vi "Calc Stat.vi"(9 "Query Parameters":T1, 11 "Channel Data":dbl[](array[numeric])) -> (0 "Maximum":dbl, 1 "Variance":dbl, 2 "Standard Deviation":dbl, 3 "Mean":dbl, 4 "Minimum":dbl, 5 "Median":dbl, 6 "N":dbl)   [LabVIEW 2011]
uses:
  Datasheet Analysis Parameters.ctl
  <vilib>/Analysis/NI_AALBase.lvlib
panel:
  # "DELAY format data must be calculated prior to passing to this VI"
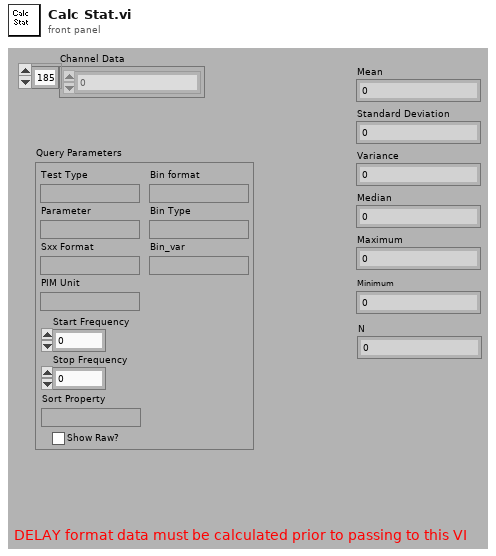
[diagram p1: front panel]
types:
  T1 = typedef "Datasheet Analysis Parameters.ctl" = cluster{"Test Type":string, "Parameter":string, "Sxx Format":string, "PIM Unit":string, "Start Frequency":dbl, "Stop Frequency":dbl, "Sort Property":string, "Show Raw?":bool, "Bin format":string, "Bin Type":string, "Bin_var":string}
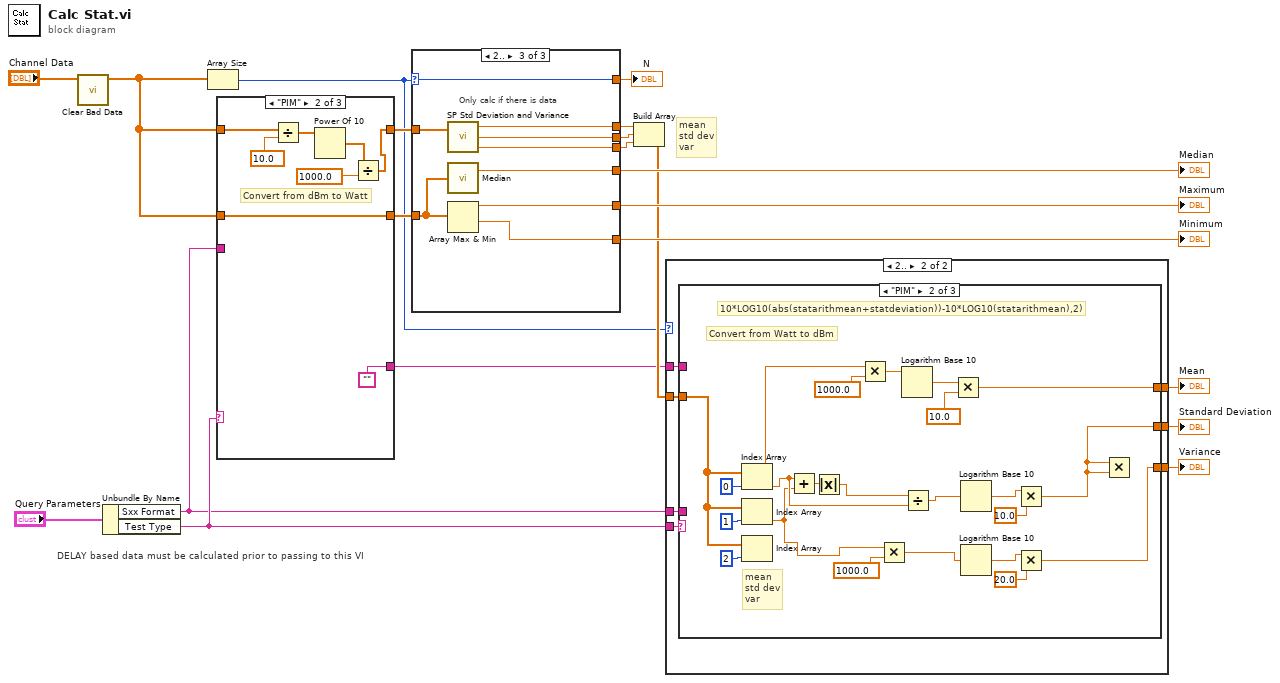
[diagram p0: block diagram]
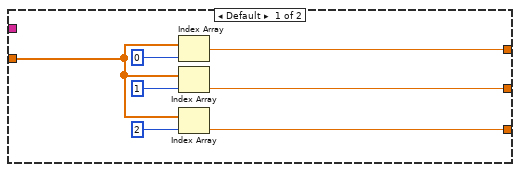
[diagram p2: hidden frame]
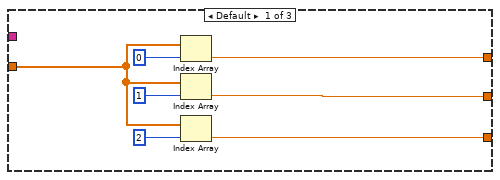
[diagram p3: hidden frame]
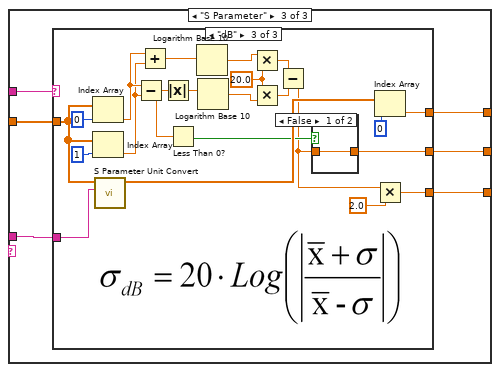
[diagram p4: hidden frame]
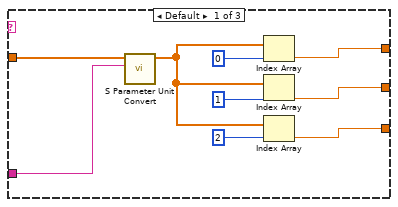
[diagram p5: hidden frame]
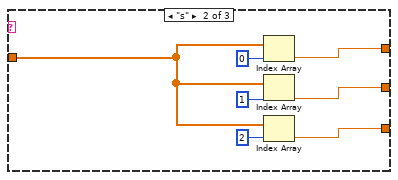
[diagram p6: hidden frame]
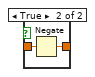
[diagram p7: hidden frame]
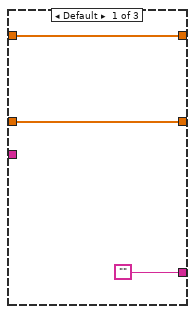
[diagram p8: hidden frame]
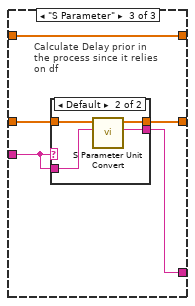
[diagram p9: hidden frame]
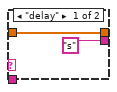
[diagram p10: hidden frame]
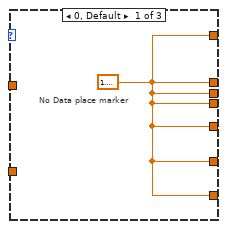
[diagram p11: hidden frame]
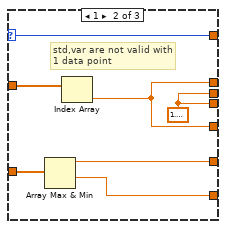
[diagram p12: hidden frame]
diagram:
  # "mean\nstd dev\nvar"
  # "DELAY based data must be calculated prior to passing to this VI"
  n1 = call "Clear Bad Data.vi"("Waveform IN"="Channel Data") -> ("Waveform out"=w3:dbl[])  [unwired: 10 out]
  n2 = Unbundle By Name("Query Parameters") -> ("Sxx Format"=w15:string, "Test Type"=w16:string)
  n3 = Array Size(array=w3) -> (size(s)=w2:i32)
  n4 = case shown="\"PIM\"" w16 {
    tunnel: w3 -> [w23 w26 w36]
    tunnel: [w23 w26 w35] -> w14
    tunnel: w15 -> [_ _ w33]
    tunnel: ["" "" w34] -> w6
    tunnel: [w21 w24 w32] -> w4
    tunnel: w3 -> [w21 w27 w32]
    frame Default {
    }
    frame "PIM" {
      # "Convert from dBm to Watt"
      n5 = Divide(x=w27, y=10.0) -> (x/y=w28:dbl[])
      n6 = Power Of 10(x=w28) -> (10^x=w29:dbl[])
      n7 = Divide(x=w29, y=1000.0) -> (x/y=w24:dbl[])
    }
    frame "S Parameter" {
      # "Calculate Delay prior in the process since it relies on df"
      n8 = case shown="Default" w33 {
        tunnel: w36 -> [w38 w42]
        tunnel: [w38 w41] -> w35
        tunnel: w33 -> [_ w40]
        tunnel: ["s" w39] -> w34
        frame "delay" {
        }
        frame Default {
          n9 = call "S Parameter Unit Convert.vi"("Format"=w40, "Waveform IN"=w42) -> ("Units"=w39:string, "Waveform out"=w41:dbl[])  [unwired: 1 in, 7 out]
        }
      }
    }
  }
  n10 = case shown="2.." w2 {
    selector: w2 -> [_ w44 w53]
    tunnel: [w43 w45 w59] -> w19
    tunnel: [w43 w47 w58] -> w18
    tunnel: [w43 w47 w57] -> w17
    tunnel: [w43 w45 w51] -> w13
    tunnel: [w43 w50 w56] -> w12
    tunnel: [w43 w49 w55] -> w11
    tunnel: w14 -> [_ w48 w52]
    tunnel: w4 -> [_ w46 w54]
    tunnel: [w43 w44 w53] -> w1
    frame 0, Default {
      w43 = 1.1447298858494002
      # "No Data place marker"
    }
    frame 1 {
      w47 = 1.1447298858494002
      # "std,var are not valid with\n1 data point"
      n11 = Array Max & Min(array=w48) -> (max value=w50:dbl, min value=w49:dbl)  [unwired: 2 out]
      n12 = Index Array(array=w46) -> (element=w45:dbl)  [unwired: 1 in]
    }
    frame 2.. {
      # "Only calc if there is data"
      n13 = call "SP Std Deviation and Variance.vi"("X"=w54) -> ("mean"=w59:dbl, "standard deviation"=w58:dbl, "variance"=w57:dbl)  [unwired: 1 in]
      n14 = call <vilib>:"Median.vi"("X"=w52) -> ("median"=w51:dbl)  [unwired: 1 out]
      n15 = Array Max & Min(array=w52) -> (max value=w56:dbl, min value=w55:dbl)  [unwired: 2 out]
    }
  }
  "Minimum" <- w11
  "Maximum" <- w12
  "Median" <- w13
  "N" <- w1
  n16 = Build Array(w19, w18, w17) -> (w9:dbl[])
  n17 = case shown="2.." w2 {
    tunnel: w16 -> [_ w73]
    tunnel: w15 -> [_ w72]
    tunnel: w9 -> [w63 w71]
    tunnel: [w62 w70] -> w8
    tunnel: [w60 w69] -> w7
    tunnel: w6 -> [_ w68]
    tunnel: [w61 w67] -> w5
    frame Default {
      n18 = Index Array(array=w63, index=0) -> (element=w62:dbl)
      n19 = Index Array(array=w63, index=1) -> (element=w61:dbl)
      n20 = Index Array(array=w63, index=2) -> (element=w60:dbl)
    }
    frame 2.. {
      n21 = case shown="\"PIM\"" w73 {
        tunnel: w71 -> [w77 w95 w108]
        tunnel: w72 -> [_ _ w107]
        tunnel: [w76 w94 w105] -> w70
        tunnel: [w75 w88 w104] -> w67
        tunnel: [w74 w85 w103] -> w69
        tunnel: w68 -> [_ _ w106]
        frame Default {
          n22 = Index Array(array=w77, index=0) -> (element=w76:dbl)
          n23 = Index Array(array=w77, index=1) -> (element=w75:dbl)
          n24 = Index Array(array=w77, index=2) -> (element=w74:dbl)
        }
        frame "PIM" {
          # "mean\nstd dev\nvar"
          # "10*LOG10(abs(statarithmean+statdeviation))-10*LOG10(statarithmean),2)"
          # "Convert from Watt to dBm"
          n25 = Index Array(array=w95, index=0) -> (element=w91:dbl)
          n26 = Index Array(array=w95, index=1) -> (element=w82:dbl)
          n27 = Index Array(array=w95, index=2) -> ()  [unwired: 1 out]
          n28 = Add(x=w91, y=w82) -> (x+y=w92:dbl)
          n29 = Absolute Value(x=w92) -> (abs(x)=w89:dbl)
          n30 = Multiply(x=w91, y=1000.0) -> (x*y=w101:dbl)
          n31 = Multiply(x=w82, y=1000.0) -> (x*y=w81:dbl)
          n32 = Logarithm Base 10(1:w101) -> (0:w99:dbl)
          n33 = Divide(x=w89, y=w91) -> (x/y=w84:dbl)
          n34 = Multiply(x=w99, y=10.0) -> (x*y=w94:dbl)
          n35 = Logarithm Base 10(1:w84) -> (0:w93:dbl)
          n36 = Logarithm Base 10(1:w81) -> (0:w86:dbl)
          n37 = Multiply(x=w93, y=10.0 ("index")) -> (x*y=w88:dbl)
          n38 = Multiply(x=w86, y=20.0 ("index")) -> (x*y=w85:dbl)
          n39 = Multiply(x=w88, y=w88) -> ()  [unwired: 1 out]
        }
        frame "S Parameter" {
          n40 = case shown="\"dB\"" w106 {
            tunnel: w108 -> [w110 w118 w140]
            tunnel: w107 -> [w117 _ w146]
            tunnel: [w113 w121 w144] -> w105
            tunnel: [w112 w120 w125] -> w104
            tunnel: [w111 w119 w131] -> w103
            frame Default {
              n41 = call "S Parameter Unit Convert.vi"("Format"=w117, "Waveform IN"=w110) -> ("Waveform out"=w109:dbl[])  [unwired: 1 in, 8 out]
              n42 = Index Array(array=w109, index=0) -> (element=w113:dbl)
              n43 = Index Array(array=w109, index=1) -> (element=w112:dbl)
              n44 = Index Array(array=w109, index=2) -> (element=w111:dbl)
            }
            frame "s" {
              n45 = Index Array(array=w118, index=0) -> (element=w121:dbl)
              n46 = Index Array(array=w118, index=1) -> (element=w120:dbl)
              n47 = Index Array(array=w118, index=2) -> (element=w119:dbl)
            }
            frame "dB" {
              w134 = 20.0 ("index")
              n48 = Index Array(array=w140, index=0) -> (element=w139:dbl)
              n49 = Index Array(array=w140, index=1) -> (element=w138:dbl)
              n50 = call "S Parameter Unit Convert.vi"("Format"=w146, "Waveform IN"=w140) -> ("Waveform out"=w143:dbl[])  [unwired: 1 in, 8 out]
              n51 = Subtract(x=w139, y=w138) -> (x-y=w128:dbl)
              n52 = Add(x=w139, y=w138) -> (x+y=w137:dbl)
              n53 = Absolute Value(x=w128) -> (abs(x)=w129:dbl)
              n54 = Less Than 0?(x=w128) -> (x < 0?=w127:bool)
              n55 = Logarithm Base 10(1:w137) -> (0:w136:dbl)
              n56 = Logarithm Base 10(1:w129) -> (0:w135:dbl)
              n57 = Multiply(x=w136, y=w134) -> (x*y=w133:dbl)
              n58 = Multiply(x=w134, y=w135) -> (x*y=w132:dbl)
              n59 = Subtract(x=w133, y=w132) -> (x-y=w126:dbl)
              n60 = case shown="False" w127 {
                tunnel: w126 -> [w147 w149]
                tunnel: [w147 w148] -> w125
                frame False {
                }
                frame True {
                  n61 = Negate(x=w149) -> (-x=w148:dbl)
                }
              }
              n62 = Index Array(array=w143, index=0) -> (element=w144:dbl)
              n63 = Multiply(x=w126, y=2.0 ("index")) -> (x*y=w131:dbl)
            }
          }
        }
      }
    }
  }
  "Variance" <- w7
  "Standard Deviation" <- w5
  "Mean" <- w8
